vi "AG33XXX.ProcEvents.vi"(0 "i ref in":refnum<vi>, 5 "error in (no error)":errorcluster) -> (14 "i ref out":refnum<vi>, 19 "error out":errorcluster)   [LabVIEW 2014, in "AG33XXX.lvlib"]
doc: "This method is used to define the events the object will listen to. Add your own events here."
uses:
  AG33XXX.lvlib
  CS_Core/BaseProcess/BaseProcess.event definition.ctl
  CS_Core/CAEObj/CAEObj.event definition.ctl
  CS_Core/BaseProcess/BaseProcess.descriptor string definition.ctl
  CS_Core/BaseProcess/BaseProcess.lvlib
  CS_Core/CAEObj/CAEObj.lvlib
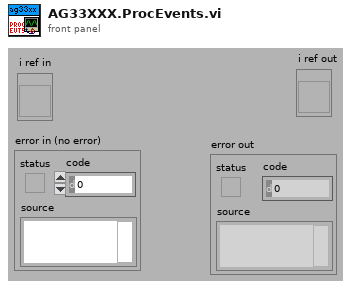
[diagram p1: front panel]
types:
  T1 = typedef "BaseProcess.lvlib/BaseProcess.event definition.ctl" = cluster{"CAEEvtDef":T2, "Data Descriptor":T3}
  T2 = typedef "CAEObj.lvlib/CAEObj.event definition.ctl" = cluster{"URL":string, "enable":bool, "ignoreResID":bool}
  T3 = typedef "BaseProcess.lvlib/BaseProcess.descriptor string definition.ctl" = string
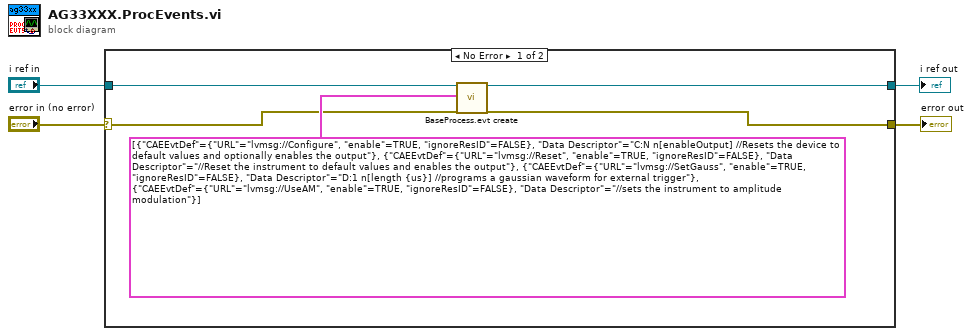
[diagram p0: block diagram]
diagram:
  n1 = case shown="No Error" "error in (no error)" {
    selector: "error in (no error)" -> [w5 w10]
    tunnel: "i ref in" -> [w9 w11]
    tunnel: [w8 w11] -> w3
    tunnel: [w7 w10] -> w2
    frame No Error {
      n2 = call "BaseProcess.evt create.vi"("i ref in"=w9, "newEvents"=T1[] [{"CAEEvtDef"={"URL"="lvmsg://Configure", "enable"=TRUE, "ignoreResID"=FALSE}, "Data Descriptor"="C:N n[enableOutput] //Resets the device to default values and optionally enables the output"}, {"CAEEvtDef"={"URL"="lvmsg://Reset", "enable"=TRUE, "ignoreResID"=FALSE}, "Data Descriptor"="//Reset the instrument to default values and enables the output"}, {"CAEEvtDef"={"URL"="lvmsg://SetGauss", "enable"=TRUE, "ignoreResID"=FALSE}, "Data Descriptor"="D:1 n[length {us}] //programs a gaussian waveform for external trigger"}, {"CAEEvtDef"={"URL"="lvmsg://UseAM", "enable"=TRUE, "ignoreResID"=FALSE}, "Data Descriptor"="//sets the instrument to amplitude modulation"}] ("new events"), "error in (no error)"=w5) -> ("i ref out"=w8:refnum<vi>, "error out"=w7:errorcluster)  [unwired: 13 in, 2 out]
    }
    frame Error {
    }
  }
  "i ref out" <- w3
  "error out" <- w2
